vi "test.vi"() -> ()   [LabVIEW 2014]
panel:
  out "iterations":i32
  out "millisecond multiple":u32
  in  "stop":bool
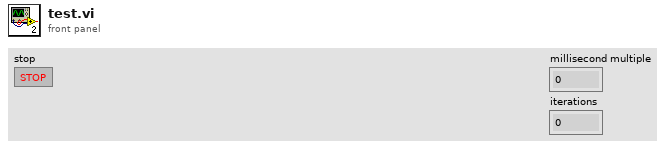
[diagram p1: front panel]
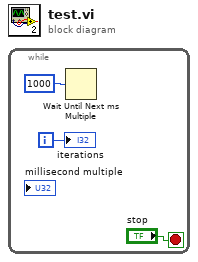
[diagram p0: block diagram]
diagram:
  n1 = while {
    i -> [w2]
    stop <- "stop" stop-if-true
    n2 = Wait Until Next ms Multiple(millisecond multiple=u32 1000) -> ()  [unwired: 1 out]
    "iterations" <- w2
  }
